vi "Test Copy Image to Pixmap No Mask ARGB.vi"(8 "error in (no error)":errorcluster, 11 "Test Case In":refnum<class "Image.lvclass">) -> (0 "error out":errorcluster, 3 "Test Case Out":refnum<class "Image.lvclass">)   [LabVIEW 2020, in "g_ar_toolkit.test.lvlib" / "Image.lvclass"]
uses:
  Image.lvclass
  C:/Program Files (x86)/National Instruments/LabVIEW 2020/vi.lib/Astemes/LUnit/Test Case.lvclass
  g_ar_toolkit.common/Image Size (Integer).ctl
  <vilib>/Astemes/LUnit/Test Case.lvclass/Test Case.ctl
  g_ar_toolkit.image/CopyImageToPixmapARGBNoMask.vi
  4993e8ee-a06a-463a-9684-69129f64d5ce.vi
  g_ar_toolkit.image/Create Image.vi
  g_ar_toolkit.image/CreateEmptyImageARGB.vi
  g_ar_toolkit.image/Copy Array to Image.vi
  g_ar_toolkit.image/CopyArrayToImageARGB.vi
  g_ar_toolkit.image/CopyImageToPixmapARGBNoMask.vi/5c639587-cf36-4d54-93d9-e654c7c24c6e.vi
  <vilib>/Astemes/LUnit/Append Pass Result.vi
  <vilib>/Astemes/LUnit/Append Fail Result.vi
  <vilib>/Astemes/LUnit/Describe Comparison.vi
  <vilib>/Astemes/LUnit/Compare Variants.vi
  g_ar_toolkit.image/CreateEmptyImageARGB.vi/3321fa97-f432-4e1e-8db9-a0df79aed21b.vi
  g_ar_toolkit.image/ARGBColourToU32.vi
  g_ar_toolkit.image/CopyArrayToImageARGB.vi/2ca5c3f0-e0c8-4997-b936-d846b6ef5cb6.vi
  <vilib>/Astemes/LUnit/Run In UI.vi
  <vilib>/Utility/error.llb/Clear Errors.vi
  g_ar_toolkit.common/Module Path.vi
  <vilib>/Utility/error.llb/Error Cluster From Error Code.vi
  <vilib>/picture/pixmap.llb/Flatten Pixmap.vi
  <vilib>/Astemes/LUnit/Describe Variant.vi
  Image.lvclass/Image.ctl
  g_ar_toolkit.common/g_ar_toolkit.common.lvlib
  g_ar_toolkit.image/g_ar_toolkit.image.lvlib
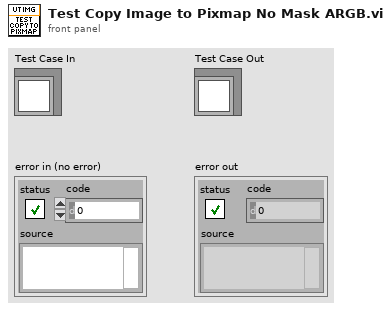
[diagram p1: front panel]
types:
  T1 = typedef "g_ar_toolkit.common.lvlib/Image Size (Integer).ctl" = cluster{"Width":u16, "Height":u16}
  T2 = typedef "imagedata.ctl" = cluster{"image type":i32, "image depth":i32, "image":u8[], "mask":u8[], "colors":u32[], "Rectangle":cluster{"left":i16, "top":i16, "right":i16, "bottom":i16}}
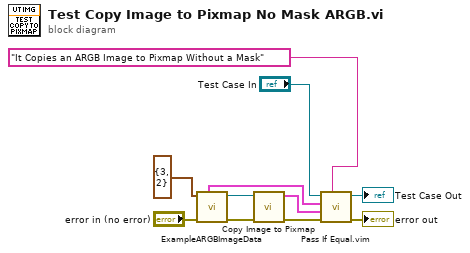
[diagram p0: block diagram]
diagram:
  n1 = call "ExampleARGBImageData.vi"("error in (no error)"="error in (no error)", "Image Size"=T1 {"Width"=3, "Height"=2} ("Preallocated Image Size (Default - 0,0)")) -> ("error out"=w7:errorcluster, "Data Value Reference out"=w4:refnum<data-value>, "ARGB Pixmap Data"=w2:T2)  [unwired: 6 in, 1 out]
  n2 = call-poly "Copy Image to Pixmap.vi"("error in (no error)"=w7, "ARGB Image Source"=w4) -> ("error out"=w3:errorcluster, "Pixmap Image Data"=w1:T2)  [unwired: 8 in]
  n3 = call "Pass If Equal.vim"("Description"="It Copies an ARGB Image to Pixmap Without a Mask", "error in (no error)"=w3, "Actual"=w1, "Expected"=w2, "LUnit Test Case In"="Test Case In") -> ("error out"=→"error out":errorcluster, "LUnit Test Case Out"=→"Test Case Out":refnum<class "Image.lvclass">)  [unwired: 5 in]
